vi "SS2 Live_Pre-Recording Checks.vi"(8 "error in (no error)":errorcluster, 9 "Init Series?":bool, 11 "SS2 Live Internal Variables in":T1={"okCFrontPanelDevices Refnum"=refnum, "Device Refnum"=refnum, "Display Image"=refnum, "# Live Images"=0, "relative s"=0.0, "# Image Sets"=0, "Message"="", "Current Image Set"=0, "# Datasets"=0, "Current Dataset"=0, "Live Mode"=FALSE, "Recording Mode"=FALSE, "Record Button"=refnum, "Live Button"=refnum, "SS2 Live Gate Data Q Name"="SS2 Live Gate Data Q", "Discard First Image"=FALSE, "Image Information"={"Save ROI Only"=FALSE, "Left"=0, "Top"=0, "Right"=0, "Bottom"=0, "Use Current ROI"=FALSE}, "Image Binning Options"={"Use Image Binning"=FALSE, "X Bin"=1, "Y Bin"=1}} {"Image Binning Options"."Y Bin" min=1; "Image Binning Options"."X Bin" min=1}) -> (0 "error out":errorcluster, 1 "Message":string, 2 "Ready?":bool, 3 "SS2 Live Internal Variables out":T1={"okCFrontPanelDevices Refnum"=refnum, "Device Refnum"=refnum, "Display Image"=refnum, "# Live Images"=0, "relative s"=0.0, "# Image Sets"=0, "Message"="", "Current Image Set"=0, "# Datasets"=0, "Current Dataset"=0, "Live Mode"=FALSE, "Recording Mode"=FALSE, "Record Button"=refnum, "Live Button"=refnum, "SS2 Live Gate Data Q Name"="SS2 Live Gate Data Q", "Discard First Image"=FALSE, "Image Information"={"Save ROI Only"=FALSE, "Left"=0, "Top"=0, "Right"=0, "Bottom"=0, "Use Current ROI"=FALSE}, "Image Binning Options"={"Use Image Binning"=FALSE, "X Bin"=1, "Y Bin"=1}} {"Image Binning Options"."Y Bin" min=1; "Image Binning Options"."X Bin" min=1}, 4 "Verbose Message":string)   [LabVIEW 2019]
uses:
  SS2 Live Internal Variables.ctl
  C:/UCLA Thinkpad Google Drive/LabVIEW 2019 SP1/builds/SS2 Live Distribution/Opal Kelly/C# Wrapper/libFrontPanel-csharp.dll
  Opal Kelly/C# Wrapper/libFrontPanel-csharp.dll
  <vilib>/vision/Image Controls.llb/IMAQ Image.ctl
  SS2 Live_Image ROI Information.ctl
  Phasor/Image Binning Options.ctl
  SS2 Live_Settings List.ctl
  SS2 Live_File Information.ctl
  SS2 Live_Globals.vi
  Variant/Variant to Data/Variant to Data.lvlib
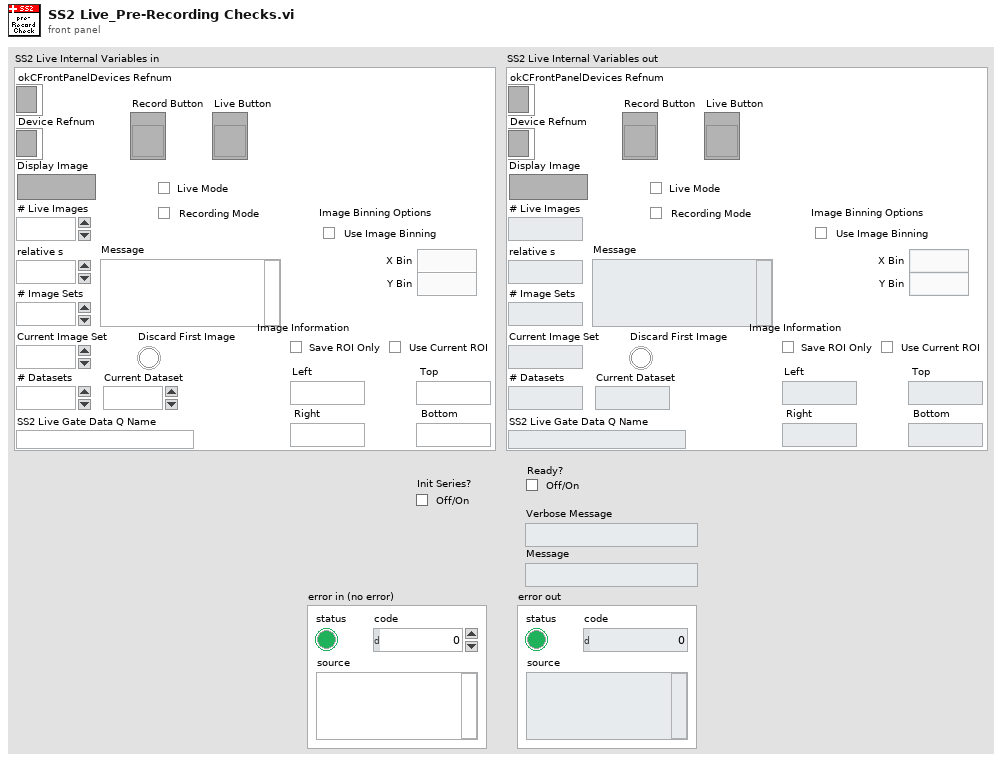
[diagram p1: front panel]
types:
  T1 = typedef "SS2 Live Internal Variables.ctl" = cluster{"okCFrontPanelDevices Refnum":refnum<k24>, "Device Refnum":refnum<k24>, "Display Image":T2, "# Live Images":i32, "relative s":dbl, "# Image Sets":i32, "Message":string, "Current Image Set":i32, "# Datasets":i32, "Current Dataset":i32, "Live Mode":bool, "Recording Mode":bool, "Record Button":refnum<vi>, "Live Button":refnum<vi>, "SS2 Live Gate Data Q Name":string, "Discard First Image":bool, "Image Information":T3, "Image Binning Options":T4}
  T2 = typedef "IMAQ Image.ctl" = refnum<image>
  T3 = typedef "SS2 Live_Image ROI Information.ctl" = cluster{"Save ROI Only":bool, "Left":u16, "Top":u16, "Right":u16, "Bottom":u16, "Use Current ROI":bool}
  T4 = typedef "Image Binning Options.ctl" = cluster{"Use Image Binning":bool, "X Bin":i32, "Y Bin":i32}
  T5 = typedef "SS2 Live_File Information.ctl" = cluster{"File Folder":path, "File Name":string, "File Index":u32, "Author":string, "Sample":string, "Compression":bool}
  T6 = typedef "SS2 Live_Settings List.ctl" = enum16{"FPGA:Bitfile Path", "FPGA:Bitfile Version", "Acquisition Parameters:SS2 DAQ Parameters", "Acquisition Parameters:Gate Configuration Array", "Acquisition Parameters:Buffer Size (# Gates)", "File Information:File Information", "File Information:# Datasets in Series", "Image Parameters:Image ROI Information", "Image Parameters:Image Binning Options", "UI Parameters:Histogram Bins Number"}
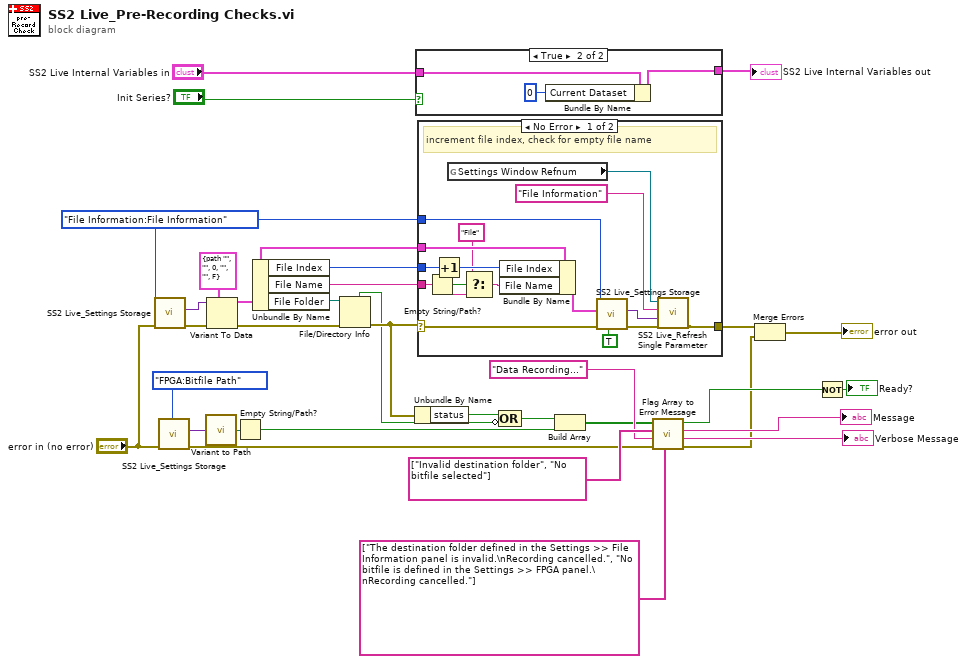
[diagram p0: block diagram]
diagram:
  w22 = SS2_Live_Settings_List."File Information:File Information" ("Settings List")
  n1 = call "SS2 Live_Settings Storage.vi"("Error In"="error in (no error)", "Settings List"=w22) -> ("Error Out"=w30:errorcluster, "Variant Data out"=w29:variant)  [unwired: 8 in]
  n2 = call "SS2 Live_Settings Storage.vi"("Error In"="error in (no error)", "Settings List"=SS2_Live_Settings_List."FPGA:Bitfile Path") -> ("Error Out"=w8:errorcluster, "Variant Data out"=w32:variant)  [unwired: 8 in]
  n3 = call "Variant to Path.vi"("Variant"=w32) -> ("Path"=w33:path)  [unwired: 8 in]
  n4 = Variant To Data(error in=w30, type=T5 {"File Folder"=path "", "File Name"="", "File Index"=0, "Author"="", "Sample"="", "Compression"=FALSE} ("File Information"), Variant=w29) -> (data=w24:T5, error out=w26:errorcluster)
  n5 = Empty String/Path?(string/path=w33) -> (empty?=w18:bool)
  n6 = Unbundle By Name(w24) -> ("File Index"=w25:u32, "File Name"=w23:string, "File Folder"=w27:path)
  n7 = File/Directory Info(path=w27, error in=w26) -> (directory=w17:bool, error out=w21:errorcluster)  [unwired: 5 out]
  n8 = Unbundle By Name(w21) -> ("status"=w19:bool)
  n9 = case shown="True" "Init Series?" {
    tunnel: "SS2 Live Internal Variables in" -> [w34 w37]
    tunnel: [w34 w36] -> w1
    frame False {
    }
    frame True {
      n10 = Bundle By Name(cluster=w37, "Current Dataset"=0) -> (w36:T1)
    }
  }
  "SS2 Live Internal Variables out" <- w1
  n11 = case shown="No Error" w21 {
    selector: w21 -> [w48 w54]
    tunnel: w25 -> [w52 _]
    tunnel: w24 -> [w53 _]
    tunnel: w23 -> [w44 _]
    tunnel: w22 -> [w49 _]
    tunnel: [w41 w54] -> w5
    frame No Error {
      # "increment file index, check for empty file name"
      n12 = Empty String/Path?(string/path=w44) -> (empty?=w46:bool)
      n13 = Increment(x=w52) -> (x+1=w51:u32)
      n14 = global read "SS2 Live_Globals.vi" "Settings Window Refnum"() -> (w40:refnum<vi>)
      n15 = Select(t="File", s=w46, f=w44) -> (s? t:f=w45:string)
      n16 = Bundle By Name(cluster=w53, "File Index"=w51, "File Name"=w45) -> (w50:T5)
      n17 = call "SS2 Live_Settings Storage.vi"("Set/Get(F)"=TRUE, "Error In"=w48, "Variant Data in"=w50, "Settings List"=w49) -> ("Error Out"=w42:errorcluster, "Variant Data out"=w39:variant)  [unwired: 6 in]
      n18 = call "SS2 Live_Refresh Single Parameter.vi"("Error In"=w42, "Data"=w39, "Control Label"="File Information", "VI Ref in"=w40) -> ("Error Out"=w41:errorcluster)  [unwired: 7 in]
    }
    frame Error {
    }
  }
  n19 = Compound Arithmetic op=OR(w19, invert w17) -> (w14:bool)
  n20 = Build Array(w14, w18) -> (w13:bool[])
  n21 = call "Flag Array to Error Message.vi"("Verbose Message Array"=string[] ["The destination folder defined in the Settings >> File Information panel is invalid.\nRecording cancelled.", "No bitfile is defined in the Settings >> FPGA panel.\nRecording cancelled."], "Error In"=w8, "OK Message"="Data Recording..." ("f"), "Message Array"=string[] ["Invalid destination folder", "No bitfile selected"], "Flag Array"=w13) -> ("Error Out"=w7:errorcluster, "Verbose Message"=→"Verbose Message":string, "Message"=→"Message":string, "Flag OR"=w9:bool)  [unwired: 3 in]
  n22 = Merge Errors(w5, w7) -> (→"error out":errorcluster)
  n23 = Not(x=w9) -> (.not. x?=→"Ready?":bool)
